vi "Process.vi"(8 "error in":errorcluster, 11 "Inst UI.RP100":refnum<class "Inst UI.RP100.lvclass">) -> (0 "error out":errorcluster, 3 "Inst UI.RP100 out":refnum<class "Inst UI.RP100.lvclass">)   [LabVIEW 2019, in "Inst.RP100.lvlib" / "Inst UI.RP100.lvclass"]
doc: "---------------------------------------------------------------\nJKI State Machine Objects™\nhttp://jki.net/state-machine-objects/\nCopyright (C) 2005-2015, JKI <info@jki.net>\nALL RIGHTS RESERVEDJKI State Machine Objects (SMO) 1.0.0.5\nJKI - JKI\nCopyright (c) 2016, JKI"
uses:
  Inst UI.RP100.lvclass
  C:/Program Files/National Instruments/LabVIEW 2019/vi.lib/JKI/JKI SMO/SMO/SMO.lvclass
  C:/Program Files/National Instruments/LabVIEW 2019/user.lib/LevyLab/Instrument Framework/Instrument UI/Instrument UI.lvclass
  C:/Program Files/National Instruments/LabVIEW 2019/vi.lib/JKI/JKI SMO/SMO.UI/SMO.UI.lvclass
  Inst.RP100/Typedefs/State--Enum.ctl
  Inst.RP100/Typedefs/Inst.RP100.getAll--Cluster.ctl
  Inst.RP100/Inst.RP100.lvclass
  C:/Program Files/National Instruments/LabVIEW 2019/user.lib/LevyLab/Instrument Framework/Instrument/Instrument.lvclass
  Inst UI.RP100.UI--Cluster.ctl
  Inst.RP100/Typedefs/Inst.RP100.Configuration--Cluster.ctl
  <userlib>/LevyLab/Configuration/Configuration.lvclass
  <userlib>/LevyLab/RemoteControl/RemoteControl/Typedefs/Message--Cluster.ctl
  <userlib>/LevyLab/Instrument Framework/Instrument UI/Instrument UI.lvclass/Instrument UI.ctl
  Inst.RP100/Inst.RP100.lvclass/Inst.RP100.ctl
  <vilib>/JKI/JKI SMO/SMO/SMO.lvclass/SMO.ctl
  <userlib>/LevyLab/Configuration/Configuration.lvclass/Configuration.ctl
  <userlib>/LevyLab/Instrument Framework/Instrument/Typedefs/Client Type--Enum.ctl
  <userlib>/LevyLab/Instrument Framework/Instrument/Instrument.lvclass/Instrument.ctl
  Inst.RP100/Typedefs/Channel--Num.ctl
  b165f17e-e592-41a1-9e74-51bdd4198767.vi
  <vilib>/JKI/JKI SMO/SMO/Private/ReftoDVR--SMO.vi
  b165f17e-e592-41a1-9e74-51bdd4198767.vi/788cc101-2700-41c1-a652-ab09bc7f8678.vi
  b165f17e-e592-41a1-9e74-51bdd4198767.vi/03a6adb6-1bef-494d-8bd2-fbb609183074.vi
  <vilib>/Utility/Data Type/Get Type Information.vi
  <vilib>/JDP Science/JSONtext/JSON text to Variant.vi
  <userlib>/LevyLab/Instrument Framework/Instrument/API/Instrument.sendMessageToProcess (variant).vi
  <userlib>/LevyLab/Instrument Framework/Instrument/Instrument.lvclass
  <vilib>/JDP Science/JSONtext/LVClass Serializer/JSONtext LVClass Serializer.lvclass
  <userlib>/LevyLab/Instrument Framework/Instrument UI/Instrument UI.lvclass
  <userlib>/LevyLab/RemoteControl/RemoteControl/RemoteControl.lvclass
  <vilib>/JKI/JKI SMO/SMO.UI/SMO.UI.lvclass
  <vilib>/JKI/JKI SMO/SMO/SMO.lvclass
  C:/Program Files/National Instruments/LabVIEW 2019/user.lib/LevyLab/Instrument Framework/Instrument Types/Strain/Instrument.Strain.lvclass
panel:
  in  "Go to Setpoint":bool
  in  "Enable Output":bool
  in  "Slew (V/s)":dbl=0.0001 min=0.0001 max=100.0 format="%#_6p"
  in  "Ch2 (V)":dbl min=-200.0 max=200.0
  in  "Ch1 (V)":dbl min=-200.0 max=200.0
  out "Ch 2 status":string="Channel 2:Shorted\n0.0V\n0.0V\n0.0V\n0.0A"
  out "Ch 1 Status":string="Channel 1:Shorted\n0.0V\n0.0V\n0.0V\n0.0A"
  out "RP100 Titles":string="RP100\nState =\nLevel =\nSlew =\nMeasured V =\nMeasured I ="
  out "Status":string="SMO State: Stopped"
  out "version":string="vDevelopment"
  # "Razorbill Monitor & Control"
  # "Actions"
  # "Setpoints"
  # "RP100 Status"
  # "SMO UI Template"
  # "For instructions on how to use the JKI State Machine Objects, examples and video tutorials, visit:\nhttp://jki.net/state-machine-objects/\n\nJKI State Machine Objects™\nhttp://jki.net/state-machine-objects/\nCopyright (C) 2005-2015, JKI <info@jki.net>\nALL RIGHTS RESERVED"
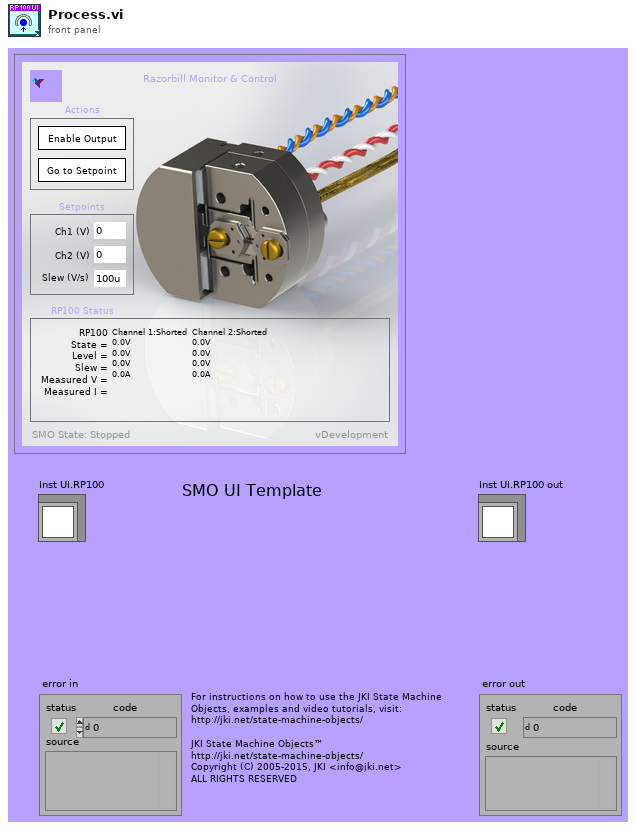
[diagram p1: front panel]
types:
  T1 = typedef "Inst.RP100.lvlib/Inst.RP100.lvclass/State--Enum.ctl" = enum16{"Shorted", "Enabled"}
  T2 = enum32{"invalid app kind", "Development System", "Run Time System", "Student Edition", "Embedded LabVIEW", "Evaluation", "Custom"}
  T3 = enum32{"Invalid", "Standard", "Closed", "Hidden", "Minimized", "Maximized"}
  T4 = typedef "Instrument.lvlib/Instrument.lvclass/Client Type--Enum.ctl" = enum16{"Remote", "Local"}
  T5 = typedef "Inst.RP100.lvlib/Inst.RP100.lvclass/Channel--Num.ctl" = i32
  T6 = typedef "RemoteControl.lvclass/Message--Cluster.ctl" = cluster{"Command":string, "Data":variant, "ID":string}
  T7 = typedef "Inst.RP100.lvlib/Inst.RP100.lvclass/Inst.RP100.Configuration--Cluster.ctl" = cluster{"Example Setting 1":dbl, "Example Setting 2":dbl, "Example Setting 3":string}
  T8 = typedef "Inst.RP100.lvlib/Inst.RP100.lvclass/Inst.RP100.getAll--Cluster.ctl" = cluster{"OutputStateCh1":string, "OutputStateCh2":string, "LevelCh1":dbl, "LevelCh2":dbl, "SlewCh1":dbl, "SlewCh2":dbl, "MeasuredVCh1":dbl, "MeasuredVCh2":dbl, "MeasuredICh1":dbl, "MeasuredICh2":dbl}
  T9 = typedef "Inst.RP100.lvlib/Inst UI.RP100.lvclass/Inst UI.RP100.UI--Cluster.ctl" = cluster{"Ch1 (V)":dbl, "Ch2 (V)":dbl, "Slew (V/s)":dbl}
  T10 = typedef "RemoteControl.lvlib/RemoteControl.lvclass/Message--Cluster.ctl" = cluster{"Command":string, "Data":variant, "ID":string}
  T11 = cluster{"Core":cluster{"Current VI Reference":refnum<vi>, "Close Panel on Exit?":bool, "Last Error":cluster{"error":errorcluster, "previous state":string, "remaining states":string}, "Shutdown?":bool}, "Instrument UI":refnum<class "Inst UI.RP100.lvclass">, "Instrument":refnum<class "Inst.RP100.lvclass">, "Configuration":refnum<class "Configuration.lvclass">, "Config Cluster":T7, "getAll":T8, "UI Cluster":T9, "Message":T10}
  T12 = typedef "SMO.lvclass/SMOState --Enum.ctl" = enum16{"unknown", "Created", "Started", "Stopped"}
  T13 = cluster{"Current VI Reference":refnum<vi>, "Close Panel on Exit?":bool, "Last Error":cluster{"error":errorcluster, "previous state":string, "remaining states":string}, "Shutdown?":bool}
  T14 = typedef "SMO.lvclass/Protected Events.ctl" = cluster{"StopProcesses":refnum<user-event>, "AbortProcesses":refnum<user-event>, "Config Changed":refnum<user-event>, "Dependency":refnum<user-event>}
  T15 = typedef "Instrument.lvlib/Instrument.lvclass/PublicEvents--Cluster.ctl" = cluster{"MessageFromProcess":refnum<user-event>}
  T16 = typedef "Inst.RP100.lvlib/Inst.RP100.lvclass/PublicEvents--Cluster.ctl" = cluster{"MessageFromProcess":refnum<user-event>}
  T17 = typedef "SMO.lvclass/Public Events.ctl" = cluster{"Error":refnum<user-event>, "State":refnum<user-event>, "Reserve State":refnum<user-event>}
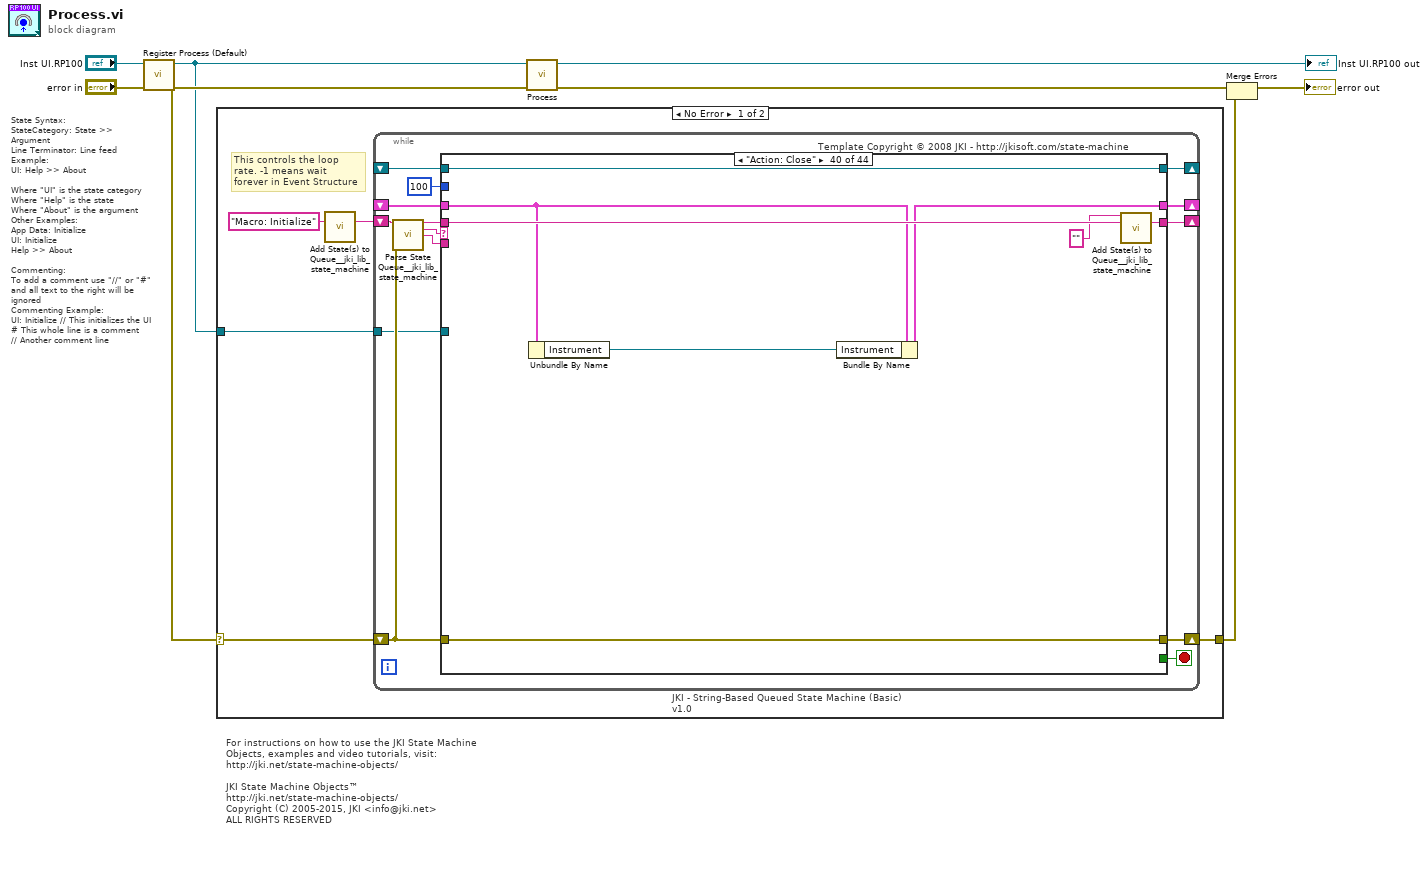
[diagram p0: block diagram]
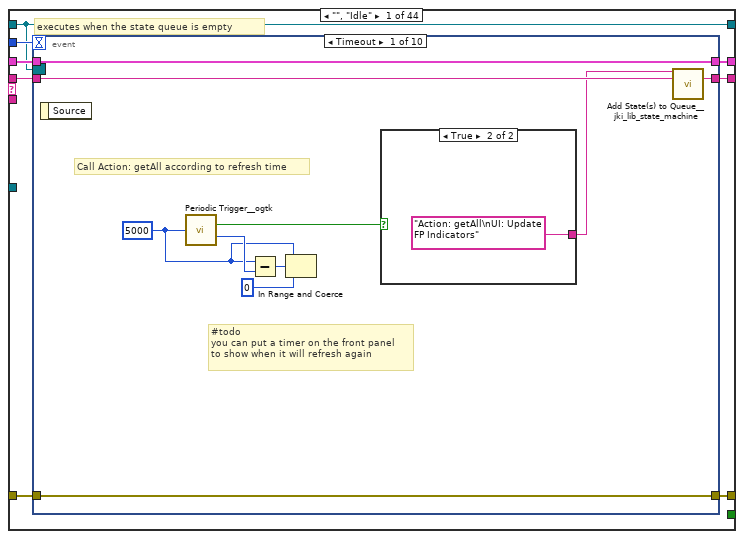
[diagram p2: hidden frame]
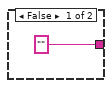
[diagram p3: hidden frame]
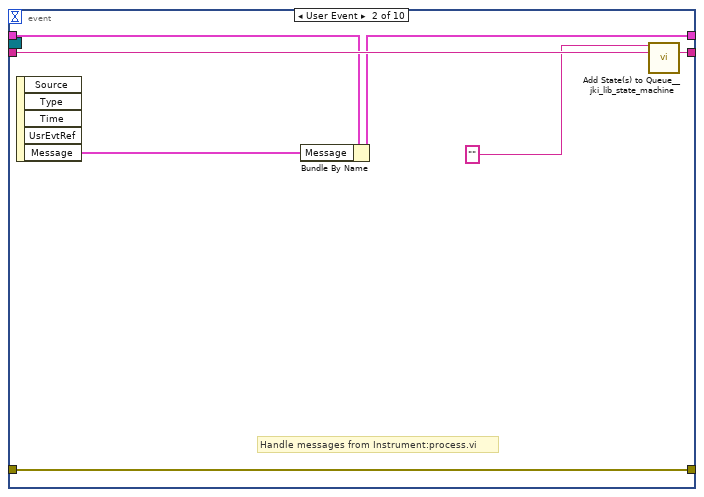
[diagram p4: hidden frame]
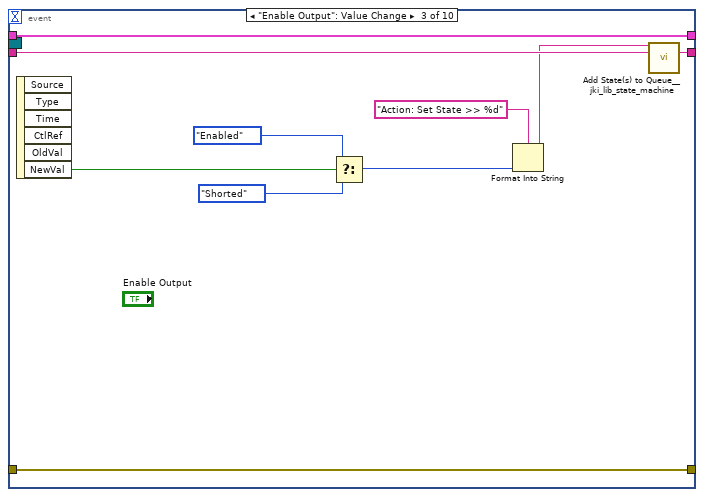
[diagram p5: hidden frame]
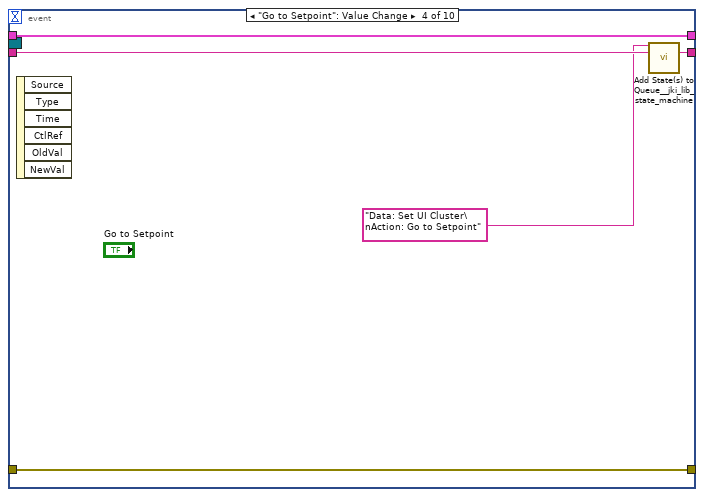
[diagram p6: hidden frame]
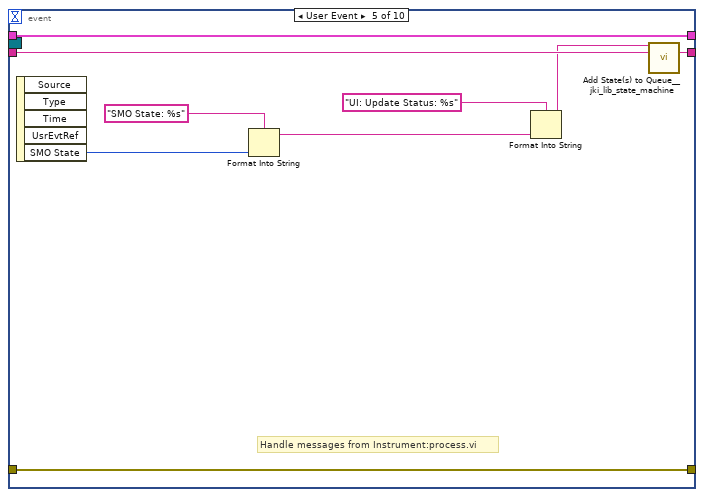
[diagram p7: hidden frame]
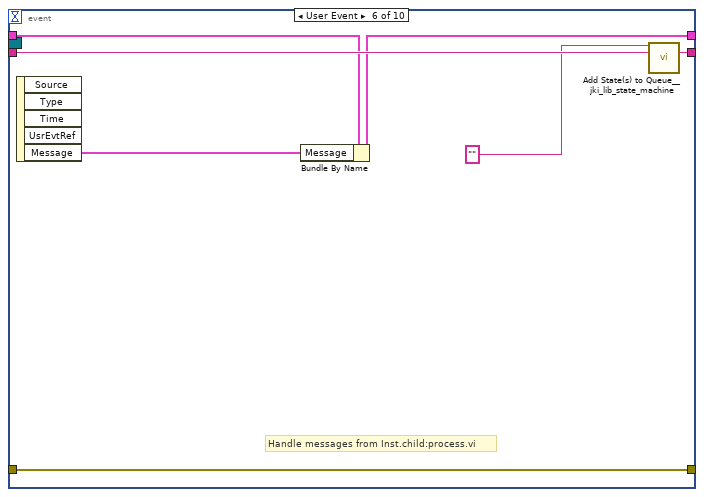
[diagram p8: hidden frame]
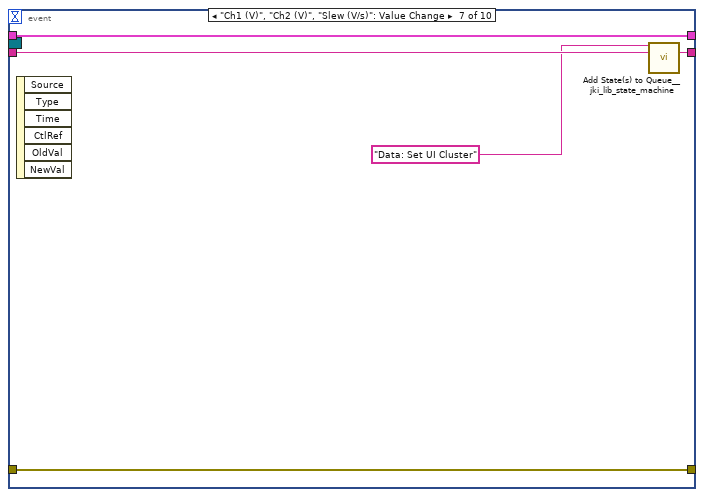
[diagram p9: hidden frame]
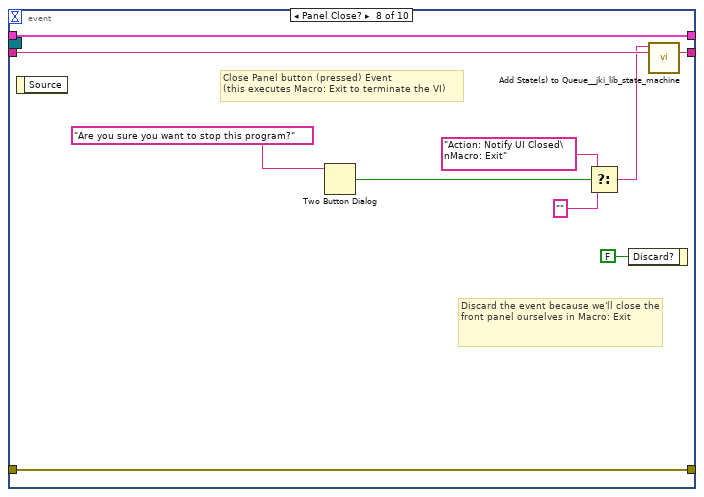
[diagram p10: hidden frame]
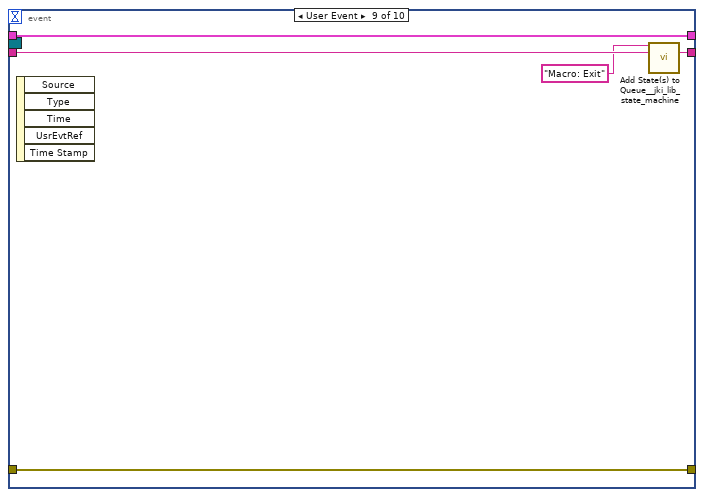
[diagram p11: hidden frame]
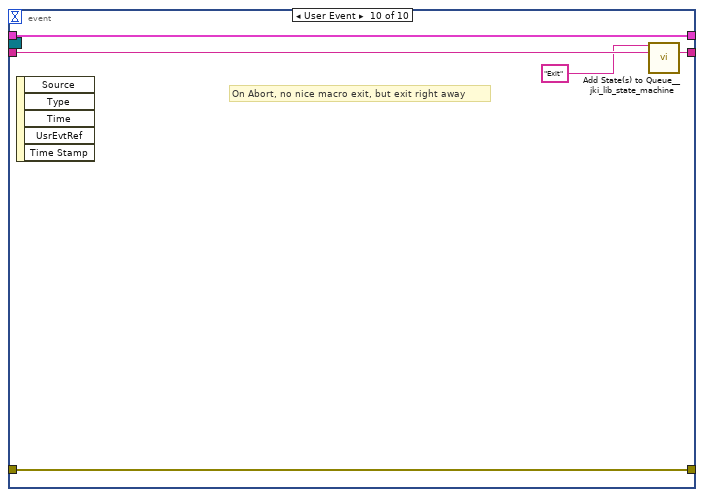
[diagram p12: hidden frame]
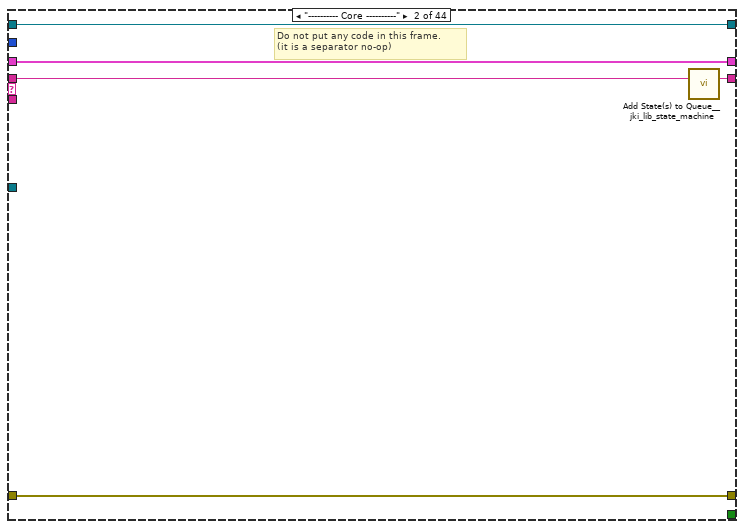
[diagram p13: hidden frame]
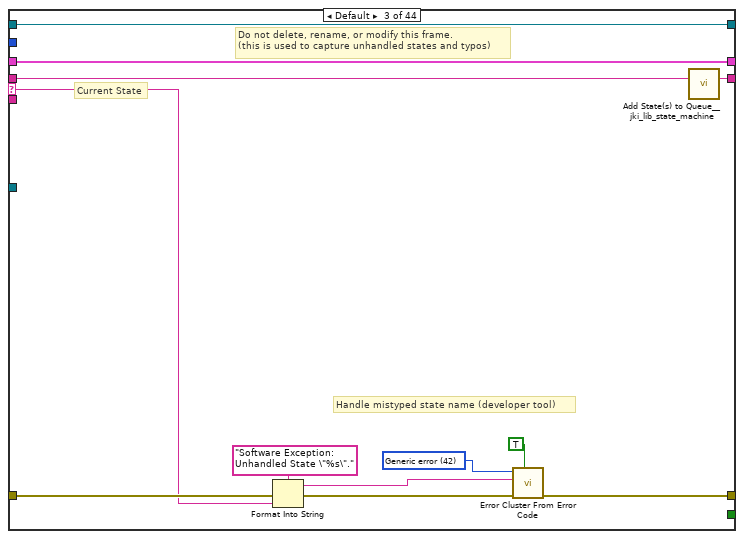
[diagram p14: hidden frame]
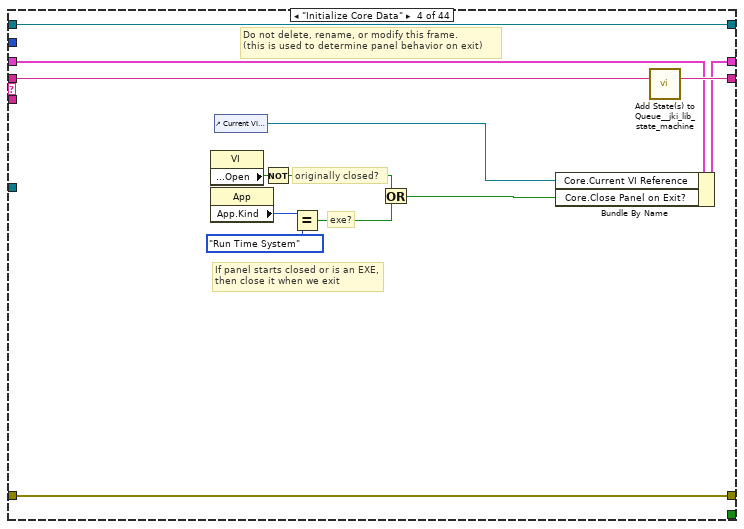
[diagram p15: hidden frame]
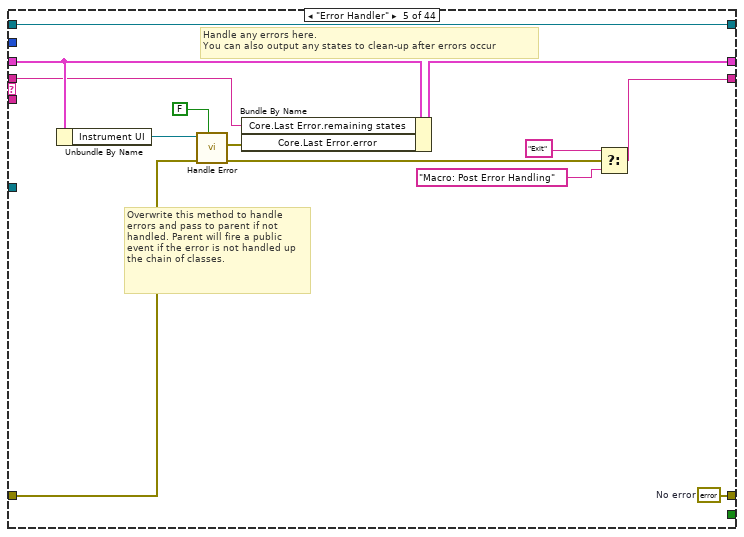
[diagram p16: hidden frame]
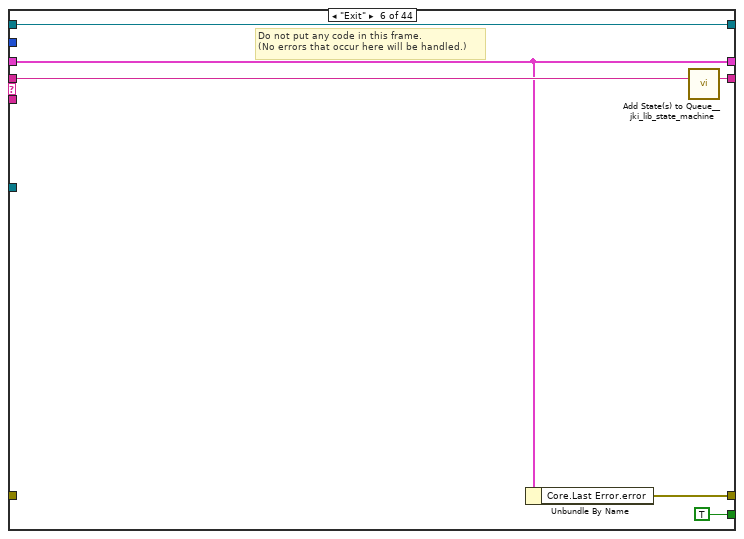
[diagram p17: hidden frame]
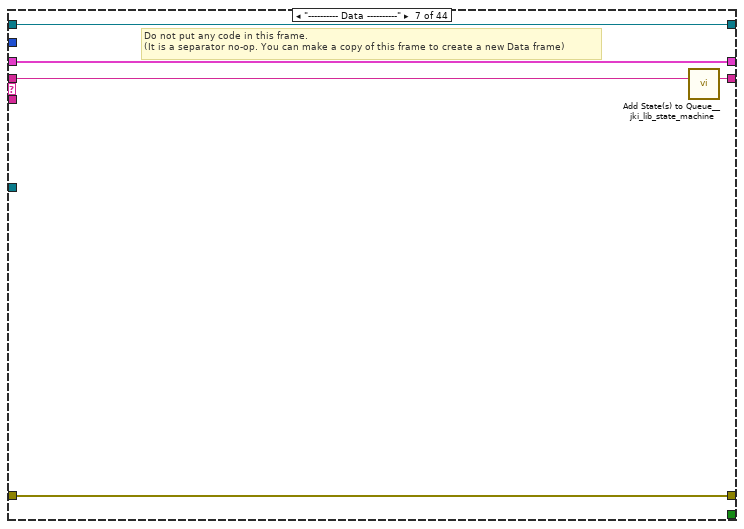
[diagram p18: hidden frame]
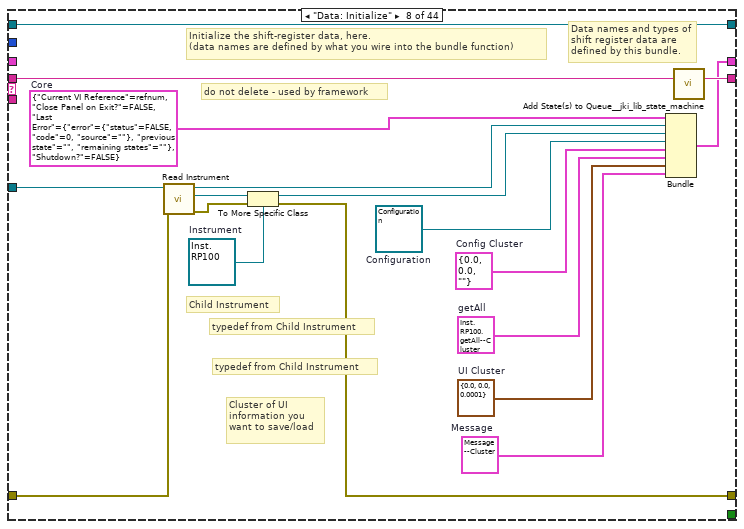
[diagram p19: hidden frame]
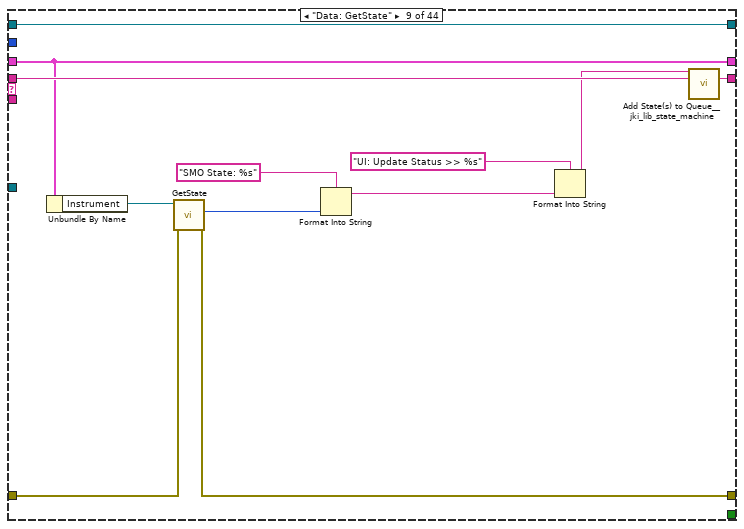
[diagram p20: hidden frame]
diagram:
  # "State Syntax:\nStateCategory: State >> Argument\nLine Terminator: Line feed\nExample:\nUI: Help >> About\n\nWhere \"UI\" is the state category\nWhere \"Help\" is the state\nWhere \"About\" is the argument\nOther Examples:\nApp Data: Initialize\nUI: Initialize\nHelp >> About\n\nCommenting:\nTo add a comment use \"//\" or \"#\" and all text to the right will be ignored\nCommenting Example:\nUI: Initialize // This initializes the UI\n# This whole line is a comment\n// Another comment line"
  # "For instructions on how to use the JKI State Machine Objects, examples and video tutorials, visit:\nhttp://jki.net/state-machine-objects/\n\nJKI State Machine Objects™\nhttp://jki.net/state-machine-objects/\nCopyright (C) 2005-2015, JKI <info@jki.net>\nALL RIGHTS RESERVED"
  n1 = call <vilib>:"Register Process (Default).vi"("error in (no error)"="error in", "SMO"="Inst UI.RP100") -> ("error out"=w5:errorcluster, "SelfRef"=w4:refnum<class "Inst UI.RP100.lvclass">)  [unwired: 8 in]
  n2 = case shown="No Error" w5 {
    selector: w5 -> [w10 w571]
    tunnel: w4 -> [w11 _]
    tunnel: [w9 w571] -> w1
    frame No Error {
      # "This controls the loop rate. -1 means wait forever in Event Structure"
      n3 = call <vilib>:"Add State(s) to Queue__jki_lib_state_machine.vi"("State(s) in (\"\")"="Macro: Initialize") -> ("States Out"=w13:string)  [unwired: 14 in]
      n4 = while "JKI - String-Based Queued State Machine (Basic) v1.0" {
        shift-right: [w20] -> _
        shift-left: _ -> [w19]
        shift-right: [w23] -> w9
        shift-left: w10 -> [w17]
        shift-right: [w22] -> _
        shift-left: w13 -> [w24]
        tunnel: w11 -> [w16]
        shift-right: [w15] -> _
        shift-left: _ -> [w14]
        stop <- w21 stop-if-true
        # "Template Copyright © 2008 JKI - http://jkisoft.com/state-machine"
        n5 = call <vilib>:"Parse State Queue__jki_lib_state_machine.vi"("State Queue"=w24, "Error In (no error)"=w17) -> ("Remaining States"=w26:string, "Current State"=w27:string, "Arguments"=w25:string)  [unwired: 11 in]
        n6 = case shown="\"Action: Close\"" w27 {
          selector: w27 -> [_ _ w117 _ _ _ _ _ _ _ _ _ _ _ _ _ _ _ _ _ _ _ _ _ _ _ _ _ _ _ _ _ _ _ _ _ _ _ _ _ _ _ _ _]
          tunnel: w26 -> [w35 w115 w121 w140 w144 w159 w164 w182 w194 w203 w211 w218 w223 w234 w240 w248 w269 w276 w292 w324 w333 w345 w355 w361 w378 w383 w394 w401 w406 w425 w431 w436 w451 w459 w471 w478 w485 w499 w510 w518 w532 w550 w560 w570]
          tunnel: w25 -> [_ _ _ _ _ _ _ _ _ _ _ _ _ _ w235 _ _ w270 w286 _ _ _ _ _ _ _ _ _ _ _ _ _ _ _ _ _ _ _ _ _ w522 _ _ _]
          tunnel: w19 -> [w33 w112 w119 w131 w147 w155 w161 _ w191 w199 w207 w212 w220 w232 w237 w244 w265 w274 w288 w321 w329 w335 w352 w358 w362 w380 w391 w396 w403 w423 w429 w433 w444 w456 w462 w473 w479 w494 w505 w511 w524 w536 w555 w565]
          tunnel: [w32 w113 w123 w137 w149 w154 w162 w169 w189 w201 w209 w214 w221 w229 w238 w246 w266 w271 w289 w322 w331 w343 w353 w359 w376 w381 w385 w397 w404 w420 w426 w434 w437 w454 w463 w475 w480 w487 w502 w512 w529 w539 w551 w561] -> w23
          tunnel: w17 -> [w31 w113 w122 w137 w143 _ w162 w166 w188 w201 w209 w215 w221 w230 w238 w246 w266 w272 w290 w322 w331 w343 w353 w359 w376 w381 w386 w398 w404 w410 w427 w434 w446 w452 w464 w475 w481 w492 w501 w512 w525 w540 w552 w562]
          tunnel: [w34 w114 w120 w139 w141 w158 w163 w181 w193 w202 w210 w217 w222 w233 w239 w247 w268 w275 w291 w323 w332 w344 w354 w360 w377 w382 w393 w400 w405 w424 w430 w435 w450 w458 w470 w477 w484 w498 w509 w517 w531 w549 w559 w569] -> w22
          tunnel: [_ _ _ _ _ TRUE _ _ _ _ _ _ _ _ _ _ _ _ _ _ _ _ _ _ _ _ _ _ _ _ _ _ _ _ _ _ _ _ _ _ _ _ _ _] -> w21
          tunnel: [w30 w112 w119 w138 w146 w155 w161 w180 w191 w198 w206 w212 w220 w232 w237 w244 w265 w274 w288 w321 w329 w336 w352 w358 w363 w380 w391 w396 w403 w423 w429 w433 w448 w456 w460 w472 w479 w495 w506 w513 w526 w546 w556 w566] -> w20
          tunnel: 100 ("Timeout") -> [w29 _ _ _ _ _ _ _ _ _ _ _ _ _ _ _ _ _ _ _ _ _ _ _ _ _ _ _ _ _ _ _ _ _ _ _ _ _ _ _ _ _ _ _]
          tunnel: w16 -> [_ _ _ _ _ _ _ w167 _ _ _ _ _ _ _ _ _ _ _ _ _ _ _ _ _ _ _ _ _ _ _ _ _ _ _ _ _ _ _ _ _ _ _ _]
          tunnel: [w28 w111 w116 w128 w153 w156 w160 w179 w192 w200 w208 w213 w219 w231 w236 w245 w267 w273 w285 w320 w330 w342 w351 w357 w370 w379 w392 w399 w402 w422 w428 w432 w449 w457 w469 w476 w483 w497 w508 w516 w530 w548 w558 w568] -> w15
          tunnel: w14 -> [w28 w111 w116 w128 w153 w156 w160 w179 w192 w200 w208 w213 w219 w231 w236 w245 w267 w273 w285 w320 w330 w342 w351 w357 w370 w379 w392 w399 w402 _ w428 w432 w449 w457 w469 w476 w483 w497 w508 w516 w530 w548 w558 w568]
          frame "", "Idle" {
            # "executes when the state queue is empty"
            n7 = event shown="[0] Timeout" {
              selector: w28 -> [_ _ _ _ _ _ _ _ _ _]
              dyn-events: _ -> [_ _ _ _ _ _ _ _ _ _]
              timeout: w29 -> [_ _ _ _ _ _ _ _ _ _]
              tunnel: w35 -> [w45 w54 w64 w69 w78 w85 w90 w100 w105 w110]
              tunnel: [w44 w53 w63 w68 w77 w84 w89 w99 w104 w109] -> w34
              tunnel: w33 -> [w42 w51 w61 w66 w75 w82 w86 w97 w102 w107]
              tunnel: [w43 w52 w62 w67 w76 w83 w88 w96 w103 w108] -> w32
              tunnel: w31 -> [w43 w52 w62 w67 w76 w83 w88 w96 w103 w108]
              tunnel: [w42 w50 w61 w66 w75 w81 w86 w97 w102 w107] -> w30
              event Timeout {
                w37 = u32 5000 ("time (ms)")
                # "#todo\nyou can put a timer on the front panel\nto show when it will refresh again"
                # "Call Action: getAll according to refresh time"
                n8 = event-data() -> ()  [unwired: 1 in, 1 out]
                n9 = call <userlib>:"Periodic Trigger__ogtk.vi"("time (ms)"=w37) -> ("Triggered"=w40:bool, "timer value"=w39:u32)  [unwired: 12 in, 1 out]
                n10 = Subtract(x=w37, y=w39) -> (x-y=w38:u32)
                n11 = In Range and Coerce(upper limit=w37, x=w38, lower limit=u32 0) -> ()  [unwired: 2 out]
                n12 = case shown="True" w40 {
                  tunnel: ["" ("State(s) in Front (\"\")") "Action: getAll\nUI: Update FP Indicators" ("State(s) in Front (\"\")")] -> w41
                  frame False {
                  }
                  frame True {
                  }
                }
                n13 = call <vilib>:"Add State(s) to Queue__jki_lib_state_machine.vi"("State(s) in Front (\"\")"=w41, "State(s) in (\"\")"=w45) -> ("States Out"=w44:string)  [unwired: 13 in]
              }
              event User Event {
                # "Handle messages from Instrument:process.vi"
                n14 = event-data() -> ("Message"=w48:T6)  [unwired: 1 in, 4 out]
                n15 = Bundle By Name(cluster=w51, "Message"=w48) -> (w50:T11)
                n16 = call <vilib>:"Add State(s) to Queue__jki_lib_state_machine.vi"("State(s) in Front (\"\")"="" ("State(s) in Front (\"\")"), "State(s) in (\"\")"=w54) -> ("States Out"=w53:string)  [unwired: 13 in]
              }
              event "Enable Output": Value Change {
                n17 = event-data() -> ("NewVal"=w58:bool)  [unwired: 1 in, 5 out]
                n18 = Select(t=State--Enum."Enabled" ("Output"), s=w58, f=State--Enum."Shorted" ("Output")) -> (s? t:f=w57:T1)
                n19 = Format Into String(format string="Action: Set State >> %d" ("State(s) in Front (\"\")"), w57) -> (resulting string=w55:string)  [unwired: 2 in, 1 out]
                n20 = call <vilib>:"Add State(s) to Queue__jki_lib_state_machine.vi"("State(s) in Front (\"\")"=w55, "State(s) in (\"\")"=w64) -> ("States Out"=w63:string)  [unwired: 13 in]
              }
              event "Go to Setpoint": Value Change {
                n21 = event-data() -> ()  [unwired: 1 in, 6 out]
                n22 = call <vilib>:"Add State(s) to Queue__jki_lib_state_machine.vi"("State(s) in Front (\"\")"="Data: Set UI Cluster\nAction: Go to Setpoint" ("State(s) in Front (\"\")"), "State(s) in (\"\")"=w69) -> ("States Out"=w68:string)  [unwired: 13 in]
              }
              event User Event {
                # "Handle messages from Instrument:process.vi"
                n23 = event-data() -> ("SMO State"=w73:T12)  [unwired: 1 in, 4 out]
                n24 = Format Into String(format string="SMO State: %s", w73) -> (resulting string=w72:string)  [unwired: 2 in, 1 out]
                n25 = Format Into String(format string="UI: Update Status: %s" ("State(s) in Front (\"\")"), w72) -> (resulting string=w70:string)  [unwired: 2 in, 1 out]
                n26 = call <vilib>:"Add State(s) to Queue__jki_lib_state_machine.vi"("State(s) in Front (\"\")"=w70, "State(s) in (\"\")"=w78) -> ("States Out"=w77:string)  [unwired: 13 in]
              }
              event User Event {
                # "Handle messages from Inst.child:process.vi"
                n27 = event-data() -> ("Message"=w79:T10)  [unwired: 1 in, 4 out]
                n28 = Bundle By Name(cluster=w82, "Message"=w79) -> (w81:T11)
                n29 = call <vilib>:"Add State(s) to Queue__jki_lib_state_machine.vi"("State(s) in Front (\"\")"="" ("State(s) in Front (\"\")"), "State(s) in (\"\")"=w85) -> ("States Out"=w84:string)  [unwired: 13 in]
              }
              event "Ch1 (V)", "Ch2 (V)", "Slew (V/s)": Value Change {
                n30 = event-data() -> ()  [unwired: 1 in, 6 out]
                n31 = call <vilib>:"Add State(s) to Queue__jki_lib_state_machine.vi"("State(s) in Front (\"\")"="Data: Set UI Cluster" ("State(s) in Front (\"\")"), "State(s) in (\"\")"=w90) -> ("States Out"=w89:string)  [unwired: 13 in]
              }
              event Panel Close? {
                # "Discard the event because we'll close the front panel ourselves in Macro: Exit"
                # "Close Panel button (pressed) Event\n(this executes Macro: Exit to terminate the VI)"
                n32 = event-data() -> ()  [unwired: 1 in, 1 out]
                n33 = Two Button Dialog(message="Are you sure you want to stop this program?") -> (T button?=w95:bool)  [unwired: 2 in]
                n34 = Select(t="Action: Notify UI Closed\nMacro: Exit", s=w95, f="") -> (s? t:f=w92:string)
                n35 = event-data("Discard?"=FALSE) -> ()  [unwired: 1 in, 1 out]
                n36 = call <vilib>:"Add State(s) to Queue__jki_lib_state_machine.vi"("State(s) in Front (\"\")"=w92, "State(s) in (\"\")"=w100) -> ("States Out"=w99:string)  [unwired: 13 in]
              }
              event User Event {
                n37 = event-data() -> ()  [unwired: 1 in, 5 out]
                n38 = call <vilib>:"Add State(s) to Queue__jki_lib_state_machine.vi"("State(s) in Front (\"\")"="Macro: Exit", "State(s) in (\"\")"=w105) -> ("States Out"=w104:string)  [unwired: 13 in]
              }
              event User Event {
                # "On Abort, no nice macro exit, but exit right away"
                n39 = event-data() -> ()  [unwired: 1 in, 5 out]
                n40 = call <vilib>:"Add State(s) to Queue__jki_lib_state_machine.vi"("State(s) in Front (\"\")"="Exit", "State(s) in (\"\")"=w110) -> ("States Out"=w109:string)  [unwired: 13 in]
              }
            }
          }
          frame "---------- Core ----------" {
            # "Do not put any code in this frame.\n(it is a separator no-op)"
            n41 = call <vilib>:"Add State(s) to Queue__jki_lib_state_machine.vi"("State(s) in (\"\")"=w115) -> ("States Out"=w114:string)  [unwired: 14 in]
          }
          frame Default {
            w126 = 42 items=["No error", "Argument error", "Memory is full", "Out of zone", "End of file", "File already open", "Generic file I/O error", "File not found", "File permission error", "Disk is full", "Duplicate path", "Too many files open", "System feature not enabled", "Resource file not found", "Cannot add resource", "Resource not found", "Image not found", "Image memory error", "Pen does not exist", "Config type invalid", "Config token not found", "Config parse error", "Config memory error", "Bad external code format", "Bad external code offset", "External code not present", "Null window", "Destroy window error", "Null menu", "Print aborted", "Bad print record", "Print driver error", "Windows error during printing", "Memory error during printing", "Print dialog error", "Generic print error", "Invalid device refnum", "Device not found", "Device parameter error", "Device unit error", "Cannot open device", "Device call aborted", "Generic error", "Cancelled by user", "Object ID too low", "Object ID too high", "Object not in heap", "Unknown heap", "Unknown object (invalid DefProc)", "Unknown object (DefProc not in table)", "Message out of range", "Invalid (null) method", "Unknown message", "Manager call not supported", "Bad address", "Network operation in progress", "Network operation timed out", "Connection is busy", "Network attribute not supported", "Network error", "Address in use", "System out of memory", "Connection aborted", "Connection refused", "Not connected", "Already connected", "Connection closed", "Initialization error (interapplication manager)", "Bad occurrence", "Wait on unbound occurrence handler", "Occurrence queue overflow", "Datalog type conflict", "Unused", "Unrecognized type (interapplication manager)", "Memory corrupt", "Failed to make temporary DLL", "Old CIN version", "Drag socket not found", "Failed to load drop-object", "Failed to register OLE object", "Failed to release OLE object", "Format specifier type mismatch", "Unknown format specifier", "Too few format specifiers", "Too many format specifiers", "Scan failed", "Newer CIN version", "Error converting to variant", "Runtime menu error", "Password tampered", "Variant attribute not found", "Incompatible variant data type", "Event data is not available", "Event Store is not present", "Occurrence is not found", "Event Queue is not created", "Event info is not available", "Refnum passed is NULL", "Error retrieving Class GUID", "Error retrieving CoClass GUID", "Error retrieving TypeLib GUID.", "Bad built application magic bytes.", "Specific driver is different from the specific driver associated with the Logical Name.", "There is no session opened to the class driver.", "Max Error", "MAX - Error with config objects", "MAX - Error loading configuration", "MAX - Group not supported"]
            # "Current State"
            # "Do not delete, rename, or modify this frame.\n(this is used to capture unhandled states and typos)"
            # "Handle mistyped state name (developer tool)"
            n42 = Format Into String(format string="Software Exception: Unhandled State \"%s\"." ("message"), error in=w122, w117) -> (resulting string=w125:string, error out=w124:errorcluster)  [unwired: 1 in]
            n43 = call <vilib>:"Error Cluster From Error Code.vi"("show call chain? (False)"=TRUE, "error in (no error)"=w124, "error message (\"\")"=w125, "error code (0)"=w126) -> ("error out"=w123:errorcluster)  [unwired: 5 in]
            n44 = call <vilib>:"Add State(s) to Queue__jki_lib_state_machine.vi"("State(s) in (\"\")"=w121) -> ("States Out"=w120:string)  [unwired: 14 in]
          }
          frame "Initialize Core Data" {
            # "Do not delete, rename, or modify this frame.\n(this is used to determine panel behavior on exit)"
            # "originally closed?"
            # "exe?"
            # "If panel starts closed or is an EXE, then close it when we exit"
            n45 = property class="VI"() -> ("Front Panel.Open"=w136:bool)  [unwired: 2 in, 2 out]
            n46 = property class="App"() -> ("App.Kind"=w135:T2)  [unwired: 2 in, 2 out]
            n47 = control-ref of="Current VI Reference"() -> (w129:refnum<vi>)
            n48 = Not(x=w136) -> (.not. x?=w133:bool)
            n49 = Equal?(x=w135, y=T2."Run Time System" ("Application:Kind")) -> (x = y?=w132:bool)
            n50 = Or(x=w133, y=w132) -> (x .or. y?=w130:bool)
            n51 = Bundle By Name(cluster=w131, "Core.Current VI Reference"=w129, "Core.Close Panel on Exit?"=w130) -> (w138:T11)
            n52 = call <vilib>:"Add State(s) to Queue__jki_lib_state_machine.vi"("State(s) in (\"\")"=w140) -> ("States Out"=w139:string)  [unwired: 14 in]
          }
          frame "Error Handler" {
            w149 = errorcluster {"status"=FALSE, "code"=0, "source"=""}  # No error
            # "Overwrite this method to handle errors and pass to parent if not handled. Parent will fire a public event if the error is not handled up the chain of classes."
            # "Handle any errors here.\nYou can also output any states to clean-up after errors occur"
            n53 = Unbundle By Name(w147) -> ("Instrument UI"=w152:refnum<class "Inst UI.RP100.lvclass">)
            n54 = call-dynamic "Handle Error.vi"("Stop on Unhandled Error (T)"=FALSE, "error in"=w143, "SMO"=w152) -> ("handling error"=w150:errorcluster, "Unhandled error"=w148:errorcluster)  [unwired: 6 in, 1 out]
            n55 = Bundle By Name(cluster=w147, "Core.Last Error.remaining states"=w144, "Core.Last Error.error"=w148) -> (w146:T11)
            n56 = Select(t="Exit", s=w150, f="Macro: Post Error Handling") -> (s? t:f=w141:string)
          }
          frame "Exit" {
            # "Do not put any code in this frame.\n(No errors that occur here will be handled.)"
            n57 = Unbundle By Name(w155) -> ("Core.Last Error.error"=w154:errorcluster)
            n58 = call <vilib>:"Add State(s) to Queue__jki_lib_state_machine.vi"("State(s) in (\"\")"=w159) -> ("States Out"=w158:string)  [unwired: 14 in]
          }
          frame "---------- Data ----------" {
            # "Do not put any code in this frame.\n(It is a separator no-op. You can make a copy of this frame to create a new Data frame)"
            n59 = call <vilib>:"Add State(s) to Queue__jki_lib_state_machine.vi"("State(s) in (\"\")"=w164) -> ("States Out"=w163:string)  [unwired: 14 in]
          }
          frame "Data: Initialize" {
            w165 = T10 {"Command"="", "Data"=variant, "ID"=""}  # Message
            w168 = refnum<class "Configuration.lvclass"> refnum  # Configuration
            w171 = T7 {"Example Setting 1"=0.0, "Example Setting 2"=0.0, "Example Setting 3"=""}  # Config Cluster
            w173 = T9 {"Ch1 (V)"=0.0, "Ch2 (V)"=0.0, "Slew (V/s)"=0.0001}  # UI Cluster
            w175 = refnum<class "Inst.RP100.lvclass"> refnum  # Instrument
            w177 = T8 {"OutputStateCh1"="", "OutputStateCh2"="", "LevelCh1"=0.0, "LevelCh2"=0.0, "SlewCh1"=0.0, "SlewCh2"=0.0, "MeasuredVCh1"=0.0, "MeasuredVCh2"=0.0, "MeasuredICh1"=0.0, "MeasuredICh2"=0.0}  # getAll
            w178 = T13 {"Current VI Reference"=refnum, "Close Panel on Exit?"=FALSE, "Last Error"={"error"={"status"=FALSE, "code"=0, "source"=""}, "previous state"="", "remaining states"=""}, "Shutdown?"=FALSE}  # Core
            # "typedef from Child Instrument"
            # "Cluster of UI\ninformation you\nwant to save/load"
            # "Child Instrument"
            # "typedef from Child Instrument"
            # "do not delete - used by framework"
            # "Data names and types of shift register data are defined by this bundle."
            # "Initialize the shift-register data, here.\n(data names are defined by what you wire into the bundle function)"
            n60 = call <userlib>:"Read Instrument.vi"("error in (no error)"=w166, "Instrument UI in"=w167) -> ("error out"=w172:errorcluster, "Instrument"=w174:refnum<class "Instrument.lvclass">, "Instrument UI"=w176:refnum<class "Inst UI.RP100.lvclass">)  [unwired: 7 in]
            n61 = To More Specific Class(target class=w175, reference=w174, error in=w172) -> (specific class reference=w170:refnum<class "Inst.RP100.lvclass">, error out=w169:errorcluster)
            n62 = Bundle("Core"=w178, "Instrument UI"=w176, "Instrument"=w170, "Configuration"=w168, "Config Cluster"=w171, "getAll"=w177, "UI Cluster"=w173, "Message"=w165) -> (w180:T11)  [unwired: 1 in]
            n63 = call <vilib>:"Add State(s) to Queue__jki_lib_state_machine.vi"("State(s) in (\"\")"=w182) -> ("States Out"=w181:string)  [unwired: 14 in]
          }
          frame "Data: GetState" {
            n64 = Unbundle By Name(w191) -> ("Instrument"=w190:refnum<class "Inst.RP100.lvclass">)
            n65 = call <vilib>:"GetState.vi"("error in (no error)"=w188, "SMO"=w190) -> ("error out"=w189:errorcluster, "SMO State"=w184:T12)  [unwired: 7 in, 1 out]
            n66 = Format Into String(format string="SMO State: %s", w184) -> (resulting string=w186:string)  [unwired: 2 in, 1 out]
            n67 = Format Into String(format string="UI: Update Status >> %s" ("State(s) in Front (\"\")"), w186) -> (resulting string=w183:string)  [unwired: 2 in, 1 out]
            n68 = call <vilib>:"Add State(s) to Queue__jki_lib_state_machine.vi"("State(s) in Front (\"\")"=w183, "State(s) in (\"\")"=w194) -> ("States Out"=w193:string)  [unwired: 13 in]
          }
          frame "Data: Set UI Cluster" {
            # "Do not put any code in this frame.\n(It is a separator no-op. You can make a copy of this frame to create a new Data frame)"
            n69 = Bundle By Name(cluster=w199, "UI Cluster.Ch1 (V)"="Ch1 (V)", "UI Cluster.Ch2 (V)"="Ch2 (V)", "UI Cluster.Slew (V/s)"="Slew (V/s)") -> (w198:T11)
            n70 = call <vilib>:"Add State(s) to Queue__jki_lib_state_machine.vi"("State(s) in (\"\")"=w203) -> ("States Out"=w202:string)  [unwired: 14 in]
          }
          frame "Data: Set Config Cluster" {
            # "Do not put any code in this frame.\n(It is a separator no-op. You can make a copy of this frame to create a new Data frame)"
            n71 = Unbundle By Name(w207) -> ("UI Cluster.Ch1 (V)"=w205:dbl)
            n72 = Square(x=w205) -> (x^2=w204:dbl)
            n73 = Bundle By Name(cluster=w207, "Config Cluster.Example Setting 1"=w205, "Config Cluster.Example Setting 2"=w204) -> (w206:T11)
            n74 = call <vilib>:"Add State(s) to Queue__jki_lib_state_machine.vi"("State(s) in (\"\")"=w211) -> ("States Out"=w210:string)  [unwired: 14 in]
          }
          frame "Data: Cleanup" {
            # "Cleanup any data and references, here.\n(this is called automatically, by the Macro: Exit)"
            n75 = Unbundle By Name(w212) -> ("Core.Current VI Reference"=w216:refnum<vi>)
            n76 = Close Reference(reference=w216, error in (no error)=w215) -> (error out=w214:errorcluster)
            n77 = call <vilib>:"Add State(s) to Queue__jki_lib_state_machine.vi"("State(s) in (\"\")"=w218) -> ("States Out"=w217:string)  [unwired: 14 in]
          }
          frame "---------- UI ----------" {
            # "Do not put any code in this frame.\n(It is a separator no-op. You can make a copy of this frame to create a new UI frame)"
            n78 = call <vilib>:"Add State(s) to Queue__jki_lib_state_machine.vi"("State(s) in (\"\")"=w223) -> ("States Out"=w222:string)  [unwired: 14 in]
          }
          frame "UI: Initialize" {
            # "size window to decoration box on front panel"
            # "Initialize the User Interface, here.\n(this is called automatically, by the Macro: Init)"
            n79 = call <userlib>:"MGI Get Executable Version.vi"() -> ("Version"=w227:string)  [unwired: 7 in]
            n80 = Format Into String(format string="v%s", w227) -> (resulting string=→"version":string)  [unwired: 2 in, 1 out]
            n81 = call <userlib>:"Fit VI window to Largest Dec__ogtk.vi"("error in (no error)"=w230, "border spacing (2 px)"=0) -> ("error out"=w229:errorcluster)  [unwired: 4 in, 1 out]
            n82 = call <vilib>:"Add State(s) to Queue__jki_lib_state_machine.vi"("State(s) in (\"\")"=w234) -> ("States Out"=w233:string)  [unwired: 14 in]
            "RP100 Titles" <- "\nState =\nLevel =\nSlew =\nMeasured V =\nMeasured I =" ("Status 2")
          }
          frame "UI: Update Status" {
            # "Do not put any code in this frame.\n(It is a separator no-op. You can make a copy of this frame to create a new UI frame)"
            n83 = call <vilib>:"Add State(s) to Queue__jki_lib_state_machine.vi"("State(s) in (\"\")"=w240) -> ("States Out"=w239:string)  [unwired: 14 in]
            "Status" <- w235
          }
          frame "UI: Update FP Controls" {
            # "Do not put any code in this frame.\n(It is a separator no-op. You can make a copy of this frame to create a new UI frame)"
            n84 = Unbundle By Name(w244) -> ("UI Cluster.Ch1 (V)"=w243:dbl, "UI Cluster.Ch2 (V)"=w242:dbl, "UI Cluster.Slew (V/s)"=w241:dbl)
            n85 = local write "Ch1 (V)"(w243) -> ()
            n86 = local write "Ch2 (V)"(w242) -> ()
            n87 = local write "Slew (V/s)"(w241) -> ()
            n88 = call <vilib>:"Add State(s) to Queue__jki_lib_state_machine.vi"("State(s) in (\"\")"=w248) -> ("States Out"=w247:string)  [unwired: 14 in]
          }
          frame "UI: Update FP Indicators" {
            w249 = "%s\\n%.1pV\\n%.1pV\\n%.1pV\\n%.1pA" ("format string")
            n89 = Unbundle By Name(w265) -> ("getAll"=w252:T8)
            n90 = Unbundle By Name(w252) -> ("OutputStateCh1"=w264:string, "LevelCh1"=w263:dbl, "SlewCh1"=w262:dbl, "MeasuredVCh1"=w261:dbl, "MeasuredICh1"=w260:dbl, "OutputStateCh2"=w259:string, "LevelCh2"=w258:dbl, "SlewCh2"=w257:dbl, "MeasuredVCh2"=w256:dbl, "MeasuredICh2"=w255:dbl)
            n91 = Format Into String(format string=w249, initial string="Channel 1:\n" ("Ch 1 Status"), w264, w263, w262, w261, w260) -> (resulting string=→"Ch 1 Status":string)  [unwired: 1 in, 1 out]
            n92 = Format Into String(format string=w249, initial string="Channel 2:\n" ("Ch 2 status"), w259, w258, w257, w256, w255) -> (resulting string=→"Ch 2 status":string)  [unwired: 1 in, 1 out]
            n93 = call <vilib>:"Add State(s) to Queue__jki_lib_state_machine.vi"("State(s) in (\"\")"=w269) -> ("States Out"=w268:string)  [unwired: 14 in]
          }
          frame "UI: Cursor Set" {
            # "Argument"
            # "Initialize the User Interface, here.\n(this is called automatically, by the Macro: Init)"
            n94 = disable-structure shown="Default" {
              disable-tunnel: w272 -> [w277 w280]
              disable-tunnel: [w277 w279] -> w271
              disable-tunnel: w270 -> [_ w278]
              frame condition #0 {
              }
              frame condition #1 (active) {
                n95 = case shown="\"Busy\"" w278 {
                  tunnel: w280 -> [w282 w284]
                  tunnel: [w281 w283] -> w279
                  frame "Idle", Default {
                    n96 = call <vilib>:"Unset Busy.vi"("error in (no error)"=w282) -> ("error out"=w281:errorcluster)  [unwired: 10 in]
                  }
                  frame "Busy" {
                    n97 = call <vilib>:"Set Busy.vi"("error in (no error)"=w284) -> ("error out"=w283:errorcluster)  [unwired: 9 in, 1 out]
                  }
                }
              }
            }
            n98 = call <vilib>:"Add State(s) to Queue__jki_lib_state_machine.vi"("State(s) in (\"\")"=w276) -> ("States Out"=w275:string)  [unwired: 14 in]
          }
          frame "UI: Front Panel State" {
            # "Argument"
            # "Set Front Panel Open or Closed\n(Usage: \"UI: Front Panel State >> Open|Close\")"
            n99 = Unbundle By Name(w288) -> ("Core.Current VI Reference"=w287:refnum<vi>)
            n100 = disable-structure shown="Default" {
              disable-tunnel: w290 -> [w296 w319]
              disable-tunnel: [w295 w319] -> w289
              disable-tunnel: w287 -> [w294 _]
              disable-tunnel: w286 -> [w293 _]
              frame condition #0 (active) {
                n101 = case shown="\"Close\"" w293 {
                  tunnel: w296 -> [w300 w313]
                  tunnel: [w302 w314] -> w295
                  tunnel: w294 -> [w301 w311]
                  frame "Open", Default {
                    n102 = property class="VI"(reference=w301, error in=w300) -> (reference out=w298:refnum<vi>, error out=w299:errorcluster, "FP.State"=w297:T3)
                    n103 = case shown="\"Closed\"" w297 {
                      tunnel: [w305 w308] -> w302
                      tunnel: w299 -> [w304 w308]
                      tunnel: w298 -> [w303 _]
                      frame "Closed" {
                        n104 = invoke class="VI" method="FP.Open"(reference=w303, error in=w304, "Activate"=TRUE, "State"=T3."Standard") -> (error out=w305:errorcluster)  [unwired: 1 in, 4 out]
                      }
                      frame Default {
                      }
                    }
                  }
                  frame "Close" {
                    n105 = property class="VI"(reference=w311, error in=w313) -> (reference out=w310:refnum<vi>, error out=w312:errorcluster, "FP.State"=w309:T3)
                    n106 = case shown="Default" w309 {
                      tunnel: [w315 w318] -> w314
                      tunnel: w312 -> [w315 w317]
                      tunnel: w310 -> [_ w316]
                      frame "Invalid", "Closed" {
                      }
                      frame Default {
                        n107 = invoke class="VI" method="FP.Close"(reference=w316, error in=w317) -> (error out=w318:errorcluster)  [unwired: 1 in, 2 out]
                      }
                    }
                  }
                }
              }
              frame condition #1 {
              }
            }
            n108 = call <vilib>:"Add State(s) to Queue__jki_lib_state_machine.vi"("State(s) in (\"\")"=w292) -> ("States Out"=w291:string)  [unwired: 14 in]
          }
          frame "---------- Macro ----------" {
            # "Do not put any code in this frame.\n(It is a separator no-op. You can make a copy of this frame to create a new Macro frame)"
            n109 = call <vilib>:"Add State(s) to Queue__jki_lib_state_machine.vi"("State(s) in (\"\")"=w324) -> ("States Out"=w323:string)  [unwired: 14 in]
          }
          frame "Macro: Initialize" {
            w327 = "UI: Initialize\nMacro: Read UI Config\n//UI: Front Panel State >> Open\nAction: Open\nData: GetState\nAction: getAll\nUI: Update FP Indicators"  # UI: Initialize Macro: Read UI Config //UI: Front Panel State >> Open Action: Open Data: GetState Action: getAll UI: Update FP Indicators
            # "Initialization Macro\n(This is called once, when the VI starts)"
            n110 = call <vilib>:"Add State(s) to Queue__jki_lib_state_machine.vi"("State(s) in Front (\"\")"="Data: Initialize\nInitialize Core Data\nEvents: Register", "State(s) in (\"\")"="Process: Sync", "State(s) at Back (\"\")"=w327) -> ("States Out"=w326:string)  [unwired: 12 in]
            n111 = call <vilib>:"Add State(s) to Queue__jki_lib_state_machine.vi"("State(s) in Front (\"\")"=w326, "State(s) in (\"\")"=w333) -> ("States Out"=w332:string)  [unwired: 13 in]
          }
          frame "Macro: Post Error Handling" {
            # "Clear Last Error?"
            n112 = Unbundle By Name(w335) -> ("Core.Last Error.remaining states"=w337:string, "Core.Shutdown?"=w338:bool)
            n113 = Unbundle By Name(w335) -> ("Core.Last Error.error"=w341:errorcluster)
            n114 = case shown="False" FALSE {
              tunnel: w341 -> [w349 _]
              tunnel: [w349 _] -> w340
              frame False {
              }
              frame True {
              }
            }
            n115 = case shown="False" w338 {
              tunnel: w337 -> [w346 w348]
              tunnel: [w346 w347] -> w334
              frame False {
                # "These are the remaining states (at the moment the error occured). States can be altered according to business logic."
                # "NOT SHUTTING DOWN"
              }
              frame True {
                # "Developer can decide to alter the states but should be aware that during the shutdown process, there are certain states that must be run for the SMO to properly shut itself (and this process) down. As such, one can add states to perform additional clean-ups, but should append the remaining state to be executed."
                # "SHUTTING DOWN"
                n116 = call <vilib>:"Add State(s) to Queue__jki_lib_state_machine.vi"("State(s) in (\"\")"=w348) -> ("States Out"=w347:string)  [unwired: 14 in]
              }
            }
            n117 = Bundle By Name(cluster=w335, "Core.Last Error.error"=w340) -> (w336:T11)
            n118 = call <vilib>:"Add State(s) to Queue__jki_lib_state_machine.vi"("State(s) in Front (\"\")"=w334, "State(s) in (\"\")"=w345) -> ("States Out"=w344:string)  [unwired: 13 in]
          }
          frame "Macro: Read UI Config" {
            # "Do not put any code in this frame.\n(It is a separator no-op. You can make a copy of this frame to create a new Macro frame)"
            n119 = call <vilib>:"Add State(s) to Queue__jki_lib_state_machine.vi"("State(s) in Front (\"\")"="Configuration: Initialize\nConfiguration: Read UI Config File\nUI: Update FP Controls" ("State(s) in Front (\"\")"), "State(s) in (\"\")"=w355) -> ("States Out"=w354:string)  [unwired: 13 in]
          }
          frame "Macro: Write UI Config" {
            # "Do not put any code in this frame.\n(It is a separator no-op. You can make a copy of this frame to create a new Macro frame)"
            n120 = call <vilib>:"Add State(s) to Queue__jki_lib_state_machine.vi"("State(s) in Front (\"\")"="Data: Set UI Cluster\nConfiguration: Write UI Config File" ("State(s) in Front (\"\")"), "State(s) in (\"\")"=w361) -> ("States Out"=w360:string)  [unwired: 13 in]
          }
          frame "Macro: Exit" {
            # "Exit Macro\n(This is called once, when the VI exits)"
            n121 = Unbundle By Name(w362) -> ("Core.Close Panel on Exit?"=w375:bool)
            n122 = Bundle By Name(cluster=w362, "Core.Shutdown?"=TRUE) -> (w363:T11)
            n123 = Select(t="UI: Front Panel State >> Close", s=w375, f="" ("Empty String Constant")) -> (s? t:f=w372:string)
            n124 = call <vilib>:"Add State(s) to Queue__jki_lib_state_machine.vi"("State(s) in Front (\"\")"="Data: Cleanup\nEvents: Unregister\nProcess: Self Terminate", "State(s) in (\"\")"="Process: Sync", "State(s) at Back (\"\")"="Exit") -> ("States Out"=w367:string)  [unwired: 12 in]
            n125 = call <vilib>:"Add State(s) to Queue__jki_lib_state_machine.vi"("State(s) in Front (\"\")"="Action: Close\nMacro: Write UI Config", "State(s) in (\"\")"=w372, "State(s) at Back (\"\")"=w367) -> ("States Out"=w371:string)  [unwired: 12 in]
            n126 = call <vilib>:"Add State(s) to Queue__jki_lib_state_machine.vi"("State(s) in Front (\"\")"=w371, "State(s) in (\"\")"=w378) -> ("States Out"=w377:string)  [unwired: 13 in]
          }
          frame "---------- Process ----------" {
            # "Template Separator\n(You can make a copy of, or modify, this frame)"
            n127 = call <vilib>:"Add State(s) to Queue__jki_lib_state_machine.vi"("State(s) in (\"\")"=w383) -> ("States Out"=w382:string)  [unwired: 14 in]
          }
          frame "Process: Sync" {
            n128 = Unbundle By Name(w391) -> ("Instrument UI"=w387:refnum<class "Inst UI.RP100.lvclass">)
            n129 = call <vilib>:"WaitOnProcessSync.vi"("error in (no error)"=w386, "SMO"=w387) -> ("error out"=w385:errorcluster, "Don't run?"=w390:bool)  [unwired: 7 in, 1 out]
            n130 = Select(t="Data: Cleanup\nEvents: Unregister\nExit", s=w390, f="" ("Empty String Constant")) -> (s? t:f=w384:string)
            n131 = call <vilib>:"Add State(s) to Queue__jki_lib_state_machine.vi"("State(s) in Front (\"\")"=w384, "State(s) in (\"\")"=w394) -> ("States Out"=w393:string)  [unwired: 13 in]
          }
          frame "Process: Self Terminate" {
            n132 = Unbundle By Name(w396) -> ("Instrument UI"=w395:refnum<class "Inst UI.RP100.lvclass">)
            n133 = call <vilib>:"SelfTerminate.vi"("error in (no error)"=w398, "SMO in"=w395) -> ("error out"=w397:errorcluster)  [unwired: 8 in, 1 out]
            n134 = call <vilib>:"Add State(s) to Queue__jki_lib_state_machine.vi"("State(s) in (\"\")"=w401) -> ("States Out"=w400:string)  [unwired: 14 in]
          }
          frame "---------- Events ----------" {
            # "Template Separator\n(You can make a copy of, or modify, this frame)"
            n135 = call <vilib>:"Add State(s) to Queue__jki_lib_state_machine.vi"("State(s) in (\"\")"=w406) -> ("States Out"=w405:string)  [unwired: 14 in]
          }
          frame "Events: Register" {
            # "Expand to add\nmore events"
            # "Base Class Protected Events"
            n136 = Unbundle By Name(w423) -> ("Instrument UI"=w416:refnum<class "Inst UI.RP100.lvclass">, "Instrument"=w415:refnum<class "Inst.RP100.lvclass">)
            n137 = call <vilib>:"GetProtectedEvents.vi"("SMO"=w416) -> ("error out"=w419:errorcluster, "SMO Protected Events"=w421:T14)  [unwired: 8 in, 1 out]
            n138 = call <userlib>:"Instrument.GetPublicEvents.vi"("Instrument"=w415) -> ("error out"=w417:errorcluster, "Instrument Public Events"=w418:T15, "Instrument out"=w413:refnum<class "Inst.RP100.lvclass">)  [unwired: 8 in]
            n139 = call "Inst.RP100.GetPublicEvents.vi"("Inst.RP100 in"=w413) -> ("error out"=w412:errorcluster, "Inst.RP100 Public Events"=w414:T16, "Inst.RP100 out"=w409:refnum<class "Inst.RP100.lvclass">)  [unwired: 8 in]
            n140 = call <vilib>:"GetPublicEvents.vi"("SMO"=w409) -> ("error out"=w407:errorcluster, "Public Events"=w408:T17)  [unwired: 8 in, 1 out]
            n141 = register-events(w421, w418, w414, w408) -> (reference out=w422:refnum<event-registration>, error out=w411:errorcluster)  [unwired: 2 in]
            n142 = Merge Errors(w411, w407, w412, w417, w419, w410) -> (w420:errorcluster)
            n143 = call <vilib>:"Add State(s) to Queue__jki_lib_state_machine.vi"("State(s) in (\"\")"=w425) -> ("States Out"=w424:string)  [unwired: 14 in]
          }
          frame "Events: Unregister" {
            n144 = Unregister For Events(event registration refnum=w428, error in=w427) -> (error out=w426:errorcluster)
            n145 = call <vilib>:"Add State(s) to Queue__jki_lib_state_machine.vi"("State(s) in (\"\")"=w431) -> ("States Out"=w430:string)  [unwired: 14 in]
          }
          frame "---------- Configuration ----------" {
            # "Do not put any code in this frame.\n(It is a separator no-op. You can make a copy of this frame to create a new UI frame)"
            n146 = call <vilib>:"Add State(s) to Queue__jki_lib_state_machine.vi"("State(s) in (\"\")"=w436) -> ("States Out"=w435:string)  [unwired: 14 in]
          }
          frame "Configuration: Initialize" {
            # "Do not put any code in this frame.\n(It is a separator no-op. You can make a copy of this frame to create a new UI frame)"
            n147 = Unbundle By Name(w444) -> ("Configuration"=w442:refnum<class "Configuration.lvclass">, "Instrument"=w443:refnum<class "Inst.RP100.lvclass">)
            n148 = call <vilib>:"GetName.vi"("error in (no error)"=w446, "SMO"=w443) -> ("error out"=w445:errorcluster, "Name"=w447:string)  [unwired: 6 in, 2 out]
            n149 = call <userlib>:"Default Path.vi"("error in (no error)"=w445, "Folder Name [Application Name]"=w447, "Configuration in"=w442) -> ("error out"=w438:errorcluster, "Configuration out"=w441:refnum<class "Configuration.lvclass">)  [unwired: 7 in]
            n150 = call <userlib>:"Write Section.vi"("error in (no error)"=w438, "Section"="UI", "Configuration in"=w441) -> ("error out"=w437:errorcluster, "Configuration out"=w440:refnum<class "Configuration.lvclass">)  [unwired: 7 in]
            n151 = Bundle By Name(cluster=w444, "Configuration"=w440) -> (w448:T11)
            n152 = call <vilib>:"Add State(s) to Queue__jki_lib_state_machine.vi"("State(s) in (\"\")"=w451) -> ("States Out"=w450:string)  [unwired: 14 in]
          }
          frame "Configuration: Write UI Config File" {
            # "Do not put any code in this frame.\n(It is a separator no-op. You can make a copy of this frame to create a new Data frame)"
            n153 = Unbundle By Name(w456) -> ("Configuration"=w453:refnum<class "Configuration.lvclass">, "UI Cluster"=w455:T9)
            n154 = call <userlib>:"Write Configuration.vi"("error in (no error)"=w452, "Variant"=w455, "Configuration in"=w453) -> ("error out"=w454:errorcluster)  [unwired: 7 in, 1 out]
            n155 = call <vilib>:"Add State(s) to Queue__jki_lib_state_machine.vi"("State(s) in (\"\")"=w459) -> ("States Out"=w458:string)  [unwired: 14 in]
          }
          frame "Configuration: Read UI Config File" {
            # "Do not put any code in this frame.\n(It is a separator no-op. You can make a copy of this frame to create a new UI frame)"
            n156 = Unbundle By Name(w462) -> ("UI Cluster"=w465:T9, "Configuration"=w468:refnum<class "Configuration.lvclass">)
            n157 = call <userlib>:"Read Configuration.vi"("INI Fomatted Cluster Type"=w465, "error in (no error)"=w464, "Configuration in"=w468) -> ("error out"=w467:errorcluster, "Configuration"=w466:variant)  [unwired: 6 in, 1 out]
            n158 = Variant To Data(error in=w467, type=w465, Variant=w466) -> (data=w461:T9, error out=w463:errorcluster)
            n159 = Bundle By Name(cluster=w462, "UI Cluster"=w461) -> (w460:T11)
            n160 = call <vilib>:"Add State(s) to Queue__jki_lib_state_machine.vi"("State(s) in (\"\")"=w471) -> ("States Out"=w470:string)  [unwired: 14 in]
          }
          frame "---------- Action ----------" {
            n161 = Unbundle By Name(w473) -> ("Instrument"=w474:refnum<class "Inst.RP100.lvclass">)
            n162 = Bundle By Name(cluster=w473, "Instrument"=w474) -> (w472:T11)
            n163 = call <vilib>:"Add State(s) to Queue__jki_lib_state_machine.vi"("State(s) in (\"\")"=w478) -> ("States Out"=w477:string)  [unwired: 14 in]
          }
          frame "Action: Notify UI Closed" {
            # "Notify that the UI has been closed"
            n164 = Unbundle By Name(w479) -> ("Instrument UI"=w482:refnum<class "Inst UI.RP100.lvclass">)
            n165 = call <vilib>:"Hide.vi"("error in (no error)"=w481, "SMO.UI"=w482) -> ("error out"=w480:errorcluster)  [unwired: 8 in, 1 out]
            n166 = call <vilib>:"Add State(s) to Queue__jki_lib_state_machine.vi"("State(s) in (\"\")"=w485) -> ("States Out"=w484:string)  [unwired: 14 in]
          }
          frame "Action: getAll" {
            n167 = Unbundle By Name(w494) -> ("getAll"=w490:T8, "Instrument"=w493:refnum<class "Inst.RP100.lvclass">)
            n168 = call <userlib>:"getAll.vi"("error in (no error)"=w492, "Instrument in"=w493) -> ("error out"=w488:errorcluster, "getAll"=w489:variant, "Instrument out"=w491:refnum<class "Inst.RP100.lvclass">)  [unwired: 7 in]
            n169 = call "JSON to LVtype.vim"("type"=w490, "error in (no error)"=w488, "JSON Data in"=w489) -> ("error out"=w487:errorcluster, "Data out"=w486:T8)  [unwired: 7 in]
            n170 = Bundle By Name(cluster=w494, "Instrument"=w491, "getAll"=w486) -> (w495:T11)
            n171 = call <vilib>:"Add State(s) to Queue__jki_lib_state_machine.vi"("State(s) in Front (\"\")"="" ("State(s) in Front (\"\")"), "State(s) in (\"\")"=w499) -> ("States Out"=w498:string)  [unwired: 13 in]
          }
          frame "Action: Open" {
            n172 = Unbundle By Name(w505) -> ("Instrument"=w504:refnum<class "Inst.RP100.lvclass">)
            n173 = call <userlib>:"Write Client Type.vi"("error in (no error)"=w501, "Client Type [Remote]"=Client_Type--Enum."Local" ("Client Type"), "Instrument in"=w504) -> ("error out"=w502:errorcluster, "Instrument out"=w503:refnum<class "Inst.RP100.lvclass">)  [unwired: 7 in]
            n174 = Bundle By Name(cluster=w505, "Instrument"=w503) -> (w506:T11)
            n175 = call <vilib>:"Add State(s) to Queue__jki_lib_state_machine.vi"("State(s) in Front (\"\")"="" ("State(s) in Front (\"\")"), "State(s) in (\"\")"=w510) -> ("States Out"=w509:string)  [unwired: 13 in]
          }
          frame "Action: Close" {
            n176 = Unbundle By Name(w511) -> ("Instrument"=w514:refnum<class "Inst.RP100.lvclass">)
            n177 = Bundle By Name(cluster=w511, "Instrument"=w514) -> (w513:T11)
            n178 = call <vilib>:"Add State(s) to Queue__jki_lib_state_machine.vi"("State(s) in Front (\"\")"="" ("State(s) in Front (\"\")"), "State(s) in (\"\")"=w518) -> ("States Out"=w517:string)  [unwired: 13 in]
          }
          frame "Action: Set State" {
            n179 = Unbundle By Name(w524) -> ("Instrument"=w527:refnum<class "Inst.RP100.lvclass">)
            n180 = Scan From String(format string="%d", input string=w522, default 1=State--Enum."Shorted" ("Output")) -> (output 1=w520:T1)  [unwired: 2 in, 3 out]
            n181 = call-dynamic "setState.vi"("error in (no error)"=w525, "Output"=w520, "Inst.RP100 in"=w527) -> ("error out"=w529:errorcluster, "Inst.RP100 out"=w523:refnum<class "Inst.RP100.lvclass">)  [unwired: 7 in]
            n182 = Bundle By Name(cluster=w524, "Instrument"=w523) -> (w526:T11)
            n183 = call <vilib>:"Add State(s) to Queue__jki_lib_state_machine.vi"("State(s) in Front (\"\")"="" ("State(s) in Front (\"\")"), "State(s) in (\"\")"=w532) -> ("States Out"=w531:string)  [unwired: 13 in]
          }
          frame "Action: Go to Setpoint" {
            n184 = Unbundle By Name(w536) -> ("Instrument"=w542:refnum<class "Inst.RP100.lvclass">, "UI Cluster.Ch1 (V)"=w538:dbl, "UI Cluster.Slew (V/s)"=w537:dbl)
            n185 = call-dynamic "setLevel.vi"("Output Channel"=T5 0, "error in (no error)"=w540, "Slew (V/s)"=w537, "Level (V)"=w538, "Inst.RP100 in"=w542) -> ("error out"=w545:errorcluster, "Inst.RP100 out"=w533:refnum<class "Inst.RP100.lvclass">)  [unwired: 5 in]
            n186 = Unbundle By Name(w536) -> ("UI Cluster.Ch2 (V)"=w535:dbl, "UI Cluster.Slew (V/s)"=w534:dbl)
            n187 = call-dynamic "setLevel.vi"("Output Channel"=T5 1, "error in (no error)"=w545, "Slew (V/s)"=w534, "Level (V)"=w535, "Inst.RP100 in"=w533) -> ("error out"=w539:errorcluster, "Inst.RP100 out"=w541:refnum<class "Inst.RP100.lvclass">)  [unwired: 5 in]
            n188 = Bundle By Name(cluster=w536, "Instrument"=w541) -> (w546:T11)
            n189 = call <vilib>:"Add State(s) to Queue__jki_lib_state_machine.vi"("State(s) in Front (\"\")"="" ("State(s) in Front (\"\")"), "State(s) in (\"\")"=w550) -> ("States Out"=w549:string)  [unwired: 13 in]
          }
          frame "Action: Send Message to Instrument" {
            # "Send a message (command, data, etc) to the Instrument:process.vi"
            n190 = Unbundle By Name(w555) -> ("Instrument"=w554:refnum<class "Inst.RP100.lvclass">)  [unwired: 1 out]
            n191 = call-poly <userlib>:"Instrument.sendMessageToProcess.vi"("error in (no error)"=w552, "Instrument"=w554) -> ("error out"=w551:errorcluster, "Instrument out"=w553:refnum<class "Inst.RP100.lvclass">)  [unwired: 8 in]
            n192 = Bundle By Name(cluster=w555, "Instrument"=w553) -> (w556:T11)
            n193 = call <vilib>:"Add State(s) to Queue__jki_lib_state_machine.vi"("State(s) in Front (\"\")"="" ("State(s) in Front (\"\")"), "State(s) in (\"\")"=w560) -> ("States Out"=w559:string)  [unwired: 13 in]
          }
          frame "Action: Send Message to Child" {
            # "Send a message (command, data, etc) to the Instrument.Child:process.vi"
            n194 = Unbundle By Name(w565) -> ("Instrument"=w564:refnum<class "Inst.RP100.lvclass">)  [unwired: 1 out]
            n195 = call "Inst.RP100.MessageToProcess.vi"("error in (no error)"=w562, "Inst.RP100 in"=w564) -> ("error out"=w561:errorcluster, "Inst.RP100 out"=w563:refnum<class "Inst.RP100.lvclass">)  [unwired: 8 in]
            n196 = Bundle By Name(cluster=w565, "Instrument"=w563) -> (w566:T11)
            n197 = call <vilib>:"Add State(s) to Queue__jki_lib_state_machine.vi"("State(s) in Front (\"\")"="" ("State(s) in Front (\"\")"), "State(s) in (\"\")"=w570) -> ("States Out"=w569:string)  [unwired: 13 in]
          }
        }
      }
    }
    frame Error {
    }
  }
  n198 = call-parent "Process.vi"("error in"=w5, "Instrument UI in"=w4) -> ("error out"=w2:errorcluster, "Instrument UI out"=→"Inst UI.RP100 out":refnum<class "Inst UI.RP100.lvclass">)  [unwired: 8 in]
  n199 = Merge Errors(w2, w1) -> (→"error out":errorcluster)
